vi "Find Bold Formatting.vi"(8 "error in (no error)":errorcluster, 11 "Str Refnum":refnum<vi>) -> (0 "error out":errorcluster, 1 "Length":i32[](array[numeric]), 2 "Start":i32[](array[numeric]), 3 "Str Refnum out":refnum<vi>)   [LabVIEW 2023, in "VI Properties Editor.lvlib"]
doc: "Finds where the formatting of the text of <B>Str Refnum</B> is bold."
uses:
  VI Properties Editor.lvlib
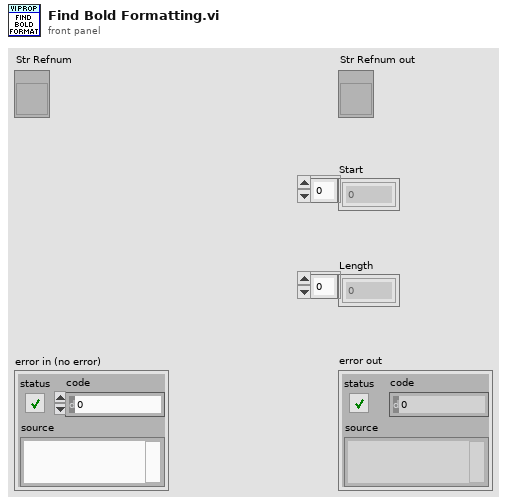
[diagram p1: front panel]
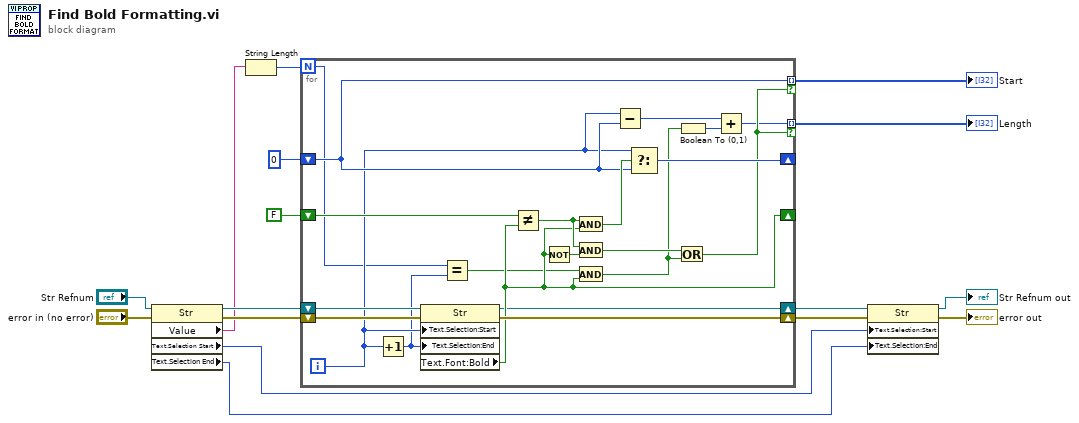
[diagram p0: block diagram]
diagram:
  n1 = property class="Str"(reference="Str Refnum", error in="error in (no error)") -> (reference out=w16:refnum<vi>, error out=w14:errorcluster, "Value"=w13:string, "Text.Selection Start"=w3:u32, "Text.Selection End"=w4:u32)
  n2 = String Length(string=w13) -> (length=w15:i32)
  n3 = for {
    N: w15 -> [w25]
    shift-right: [w26] -> _
    shift-left: FALSE -> [w35]
    shift-right: [w34] -> w6
    shift-left: w14 -> [w36]
    shift-right: [w30] -> _
    shift-left: 0 -> [w29]
    tunnel: [w29] -> w10 mode=indexing if=w22
    tunnel: [w18] -> w9 mode=indexing if=w22
    shift-right: [w17] -> w7
    shift-left: w16 -> [w37]
    i -> [w28]
    n4 = Increment(x=w28) -> (x+1=w24:i32)
    n5 = property on="Property Node" class="Str"(reference=w37, error in=w36, "Text.Selection:Start"=w28, "Text.Selection:End"=w24) -> (reference out=w17:refnum<vi>, error out=w34:errorcluster, "Text.Font:Bold"=w26:bool)
    n6 = Equal?(x=w25, y=w24) -> (x = y?=w23:bool)
    n7 = Not Equal?(x=w35, y=w26) -> (x != y?=w32:bool)
    n8 = Not(x=w26) -> (.not. x?=w31:bool)
    n9 = And(x=w32, y=w26) -> (x .and. y?=w33:bool)
    n10 = And(x=w32, y=w31) -> (x .and. y?=w27:bool)
    n11 = And(x=w23, y=w26) -> (x .and. y?=w20:bool)
    n12 = Subtract(x=w28, y=w29) -> (x-y=w21:i32)
    n13 = Select(t=w28, s=w33, f=w29) -> (s? t:f=w30:i32)
    n14 = Or(x=w27, y=w20) -> (x .or. y?=w22:bool)
    n15 = Boolean To (0,1)(Boolean=w20) -> (0, 1=w19:i16)
    n16 = Add(x=w21, y=w19) -> (x+y=w18:i32)
  }
  "Start" <- w10
  "Length" <- w9
  n17 = property on="Property Node" class="Str"(reference=w7, error in=w6, "Text.Selection:Start"=w3, "Text.Selection:End"=w4) -> (reference out=→"Str Refnum out":refnum<vi>, error out=→"error out":errorcluster)
